vi "Set_Hi-Tec_client.vi"(5 "Row No":i32=1, 6 "Strength (% by volume)":dbl format="%.2f", 7 "Carrier_2 Q (l/min)":dbl=20.0 format="%.2f", 8 "Carrier_1 Q (l/min)":dbl=20.0 format="%.2f", 9 "Mode":enum16{"Control Hi-Tec", "Check Hi-Tec Demands"}(ring)) -> (0 "error out":errorcluster, 1 "Flowrates (kg/min)":dbl[](array[numeric]) format="%.4f")   [LabVIEW 2016]
doc: "This is an example of using features of the VI Server as a client. It shows how you might browse from one or more applications that may be exporting data from one or more data stations. \n\nThe example shows how to query a server for its list of exported VIs, how to get references to the VIs, and how call them with the Call By Reference function."
uses:
  Anemometry/Anemometry Sub Vis/Globals/Preference_global.vi
panel:
  out "Iterations":i32
  in  "Server type":refnum<vi>
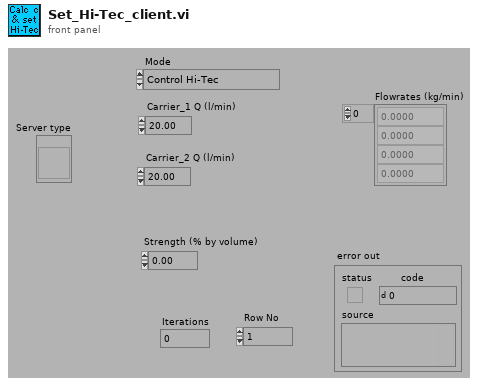
[diagram p1: front panel]
types:
  T1 = typedef "Server_Comms.ctl" = enum16{"Server Link Healthy", "Do Not Link To Server"}
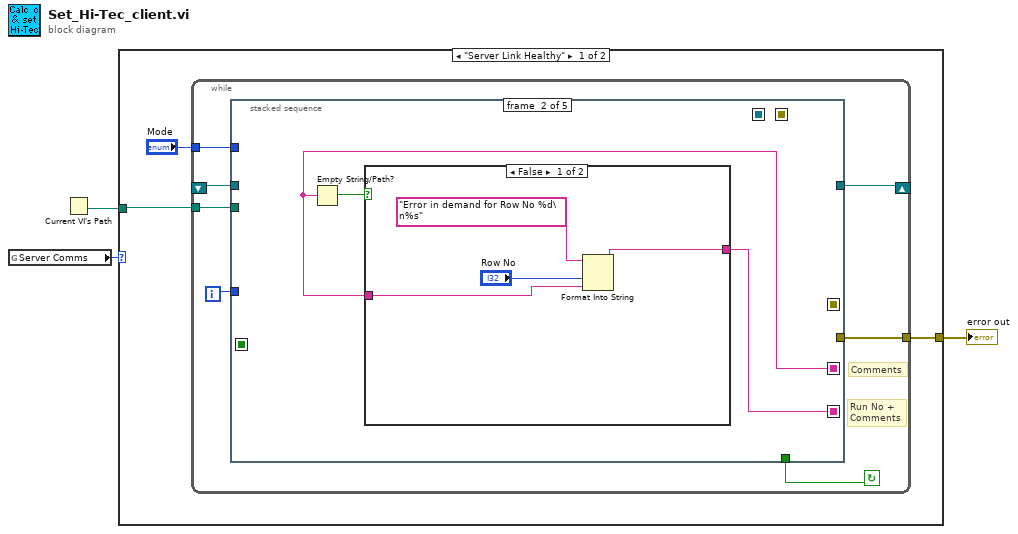
[diagram p0: block diagram]
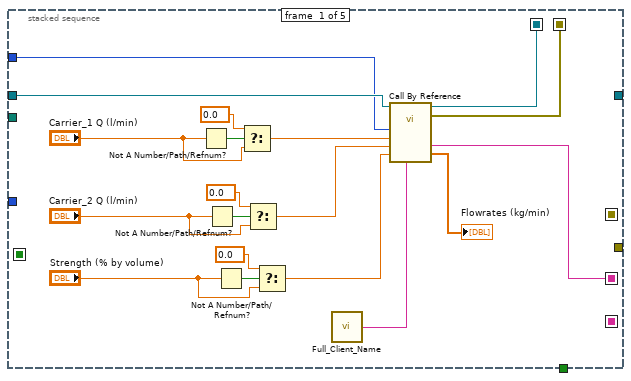
[diagram p2: hidden frame]
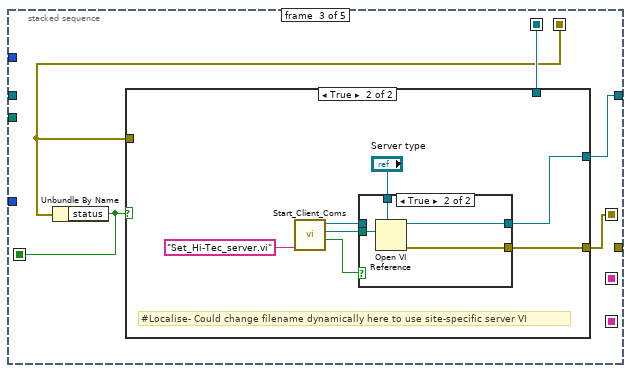
[diagram p4: hidden frame]
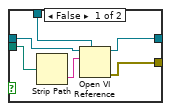
[diagram p6: hidden frame]
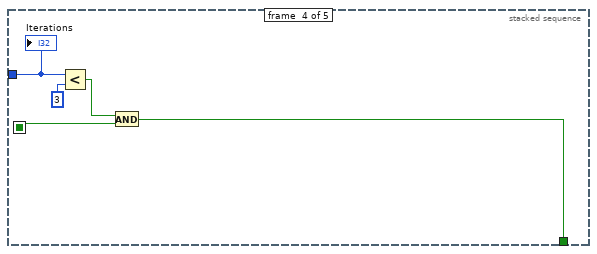
[diagram p7: hidden frame]
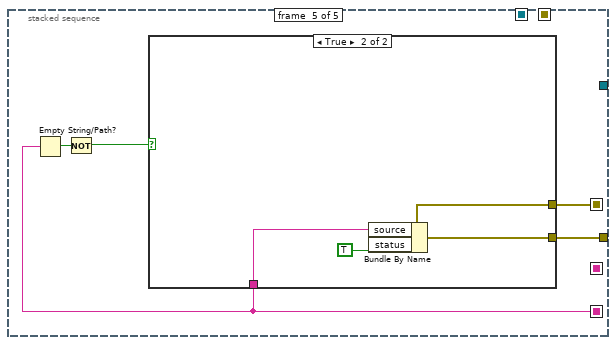
[diagram p8: hidden frame]
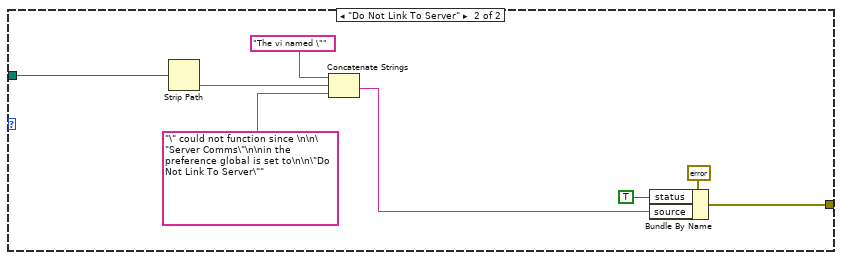
[diagram p10: hidden frame]
diagram:
  n1 = global read "Preference_global.vi" "Server Comms"() -> (w3:T1)
  n2 = Current VI's Path() -> (path=w2:path)
  n3 = case shown="\"Server Link Healthy\"" w3 {
    tunnel: [w6 w81] -> w1
    tunnel: w2 -> [w4 w80]
    frame "Server Link Healthy" {
      n4 = while {
        tunnel: w4 -> [w7]
        tunnel: "Mode" -> [w8]
        tunnel: [w9] -> w6
        shift-left: _ -> [w13]
        shift-right: [w12] -> _
        i -> [w11]
        stop <- w10 continue-if-true
        # "Run No +\nComments"
        # "Comments"
        n5 = stacked-sequence {
          seq-local: [w31 _ _ _ _] -> [_ _ w45 _ _]
          seq-local: [w30 _ _ _ _] -> [_ _ w42 _ _]
          seq-local: [_ _ w43 _ _] -> [_ _ _ w66 _]
          seq-local: [w28 _ _ _ _] -> [_ w34 _ _ _]
          seq-local: [_ w33 _ _ _] -> [_ _ _ _ w72]
          seq-local: [_ _ w41 _ _] -> [_ _ _ _ w74]
          tunnel: w13 -> [w32 _ _ _ _]
          tunnel: [_ _ w44 _ _] -> w12
          tunnel: w11 -> [_ _ _ w69 _]
          tunnel: [_ _ _ w65 _] -> w10
          tunnel: [_ _ _ _ w73] -> w9
          tunnel: w8 -> [w27 _ _ _ _]
          tunnel: w7 -> [_ _ _ _ _]
          frame #0 {
            n6 = Not A Number/Path/Refnum?(number/path/refnum="Carrier_1 Q (l/min)") -> (NaN/Path/Refnum?=w22:bool)
            n7 = Not A Number/Path/Refnum?(number/path/refnum="Carrier_2 Q (l/min)") -> (NaN/Path/Refnum?=w25:bool)
            n8 = Not A Number/Path/Refnum?(number/path/refnum="Strength (% by volume)") -> (NaN/Path/Refnum?=w18:bool)
            n9 = Select(t=0.0, s=w22, f="Carrier_1 Q (l/min)") -> (s? t:f=w16:dbl)
            n10 = Select(t=0.0, s=w25, f="Carrier_2 Q (l/min)") -> (s? t:f=w15:dbl)
            n11 = Select(t=0.0, s=w18, f="Strength (% by volume)") -> (s? t:f=w14:dbl)
            n12 = call "Full_Client_Name.vi"() -> ("Client Name"=w26:string)
            n13 = call-by-ref "?"(reference=w32, "Client Name"=w26, "Strength (% by volume)"=w14, "Carrier_2 Q (l/min)"=w15, "Carrier_1 Q (l/min)"=w16, "Mode"=w27) -> (reference out=w31:refnum<vi>, error out=w30:errorcluster, "Flowrates (kg/min)"=→"Flowrates (kg/min)":dbl[], "Comment"=w28:string)  [unwired: 4 in]
          }
          frame #1 {
            n14 = Empty String/Path?(string/path=w34) -> (empty?=w35:bool)
            n15 = case shown="False" w35 {
              tunnel: w34 -> [w36 w40]
              tunnel: [w38 w40] -> w33
              frame False {
                n16 = Format Into String(format string="Error in demand for Row No %d\n%s" ("Format String"), "Row No", w36) -> (resulting string=w38:string)  [unwired: 2 in, 1 out]
              }
              frame True {
              }
            }
          }
          frame #2 {
            n17 = Unbundle By Name(w42) -> ("status"=w43:bool)
            n18 = case shown="True" w43 {
              tunnel: w45 -> [w47 _]
              tunnel: [w47 w49] -> w44
              tunnel: [w46 w48] -> w41
              tunnel: w42 -> [w46 _]
              frame False {
              }
              frame True {
                # "#Localise- Could change filename dynamically here to use site-specific server VI"
                n19 = call "Start_Client_Coms.vi"("VI name to run on server"="Set_Hi-Tec_server.vi") -> ("LabVIEW application reference"=w53:refnum<vi>, "Checked VI name"=w54:path, "Local Call"=w52:bool)  [unwired: 1 in, 1 out]
                n20 = case shown="True" w52 {
                  tunnel: "Server type" -> [w56 w63]
                  tunnel: w54 -> [w57 w64]
                  tunnel: w53 -> [w55 _]
                  tunnel: [w59 w62] -> w49
                  tunnel: [w58 w61] -> w48
                  frame False {
                    n21 = Strip Path(path=w57) -> (name=w60:string)  [unwired: 1 out]
                    n22 = Open VI Reference(type specifier VI Refnum (for type only)=w56, application reference (local)=w55, vi path=w60) -> (vi reference=w59:refnum<vi>, error out=w58:errorcluster)  [unwired: 1 in, 2 out]
                  }
                  frame True {
                    n23 = Open VI Reference(type specifier VI Refnum (for type only)=w63, vi path=w64) -> (vi reference=w62:refnum<vi>, error out=w61:errorcluster)  [unwired: 1 in, 3 out]
                  }
                }
              }
            }
          }
          frame #3 {
            n24 = Less?(x=w69, y=3) -> (x < y?=w67:bool)
            n25 = And(x=w67, y=w66) -> (x .and. y?=w65:bool)
            "Iterations" <- w69
          }
          frame #4 {
            n26 = Empty String/Path?(string/path=w72) -> (empty?=w71:bool)
            n27 = Not(x=w71) -> (.not. x?=w70:bool)
            n28 = case shown="True" w70 {
              tunnel: w74 -> [w75 w79]
              tunnel: w72 -> [_ w76]
              tunnel: [w75 w78] -> w73
              frame False {
              }
              frame True {
                n29 = Bundle By Name(cluster=w79, "source"=w76, "status"=TRUE ("Bundle Element")) -> (w78:errorcluster)
              }
            }
          }
        }
      }
    }
    frame "Do Not Link To Server" {
      n30 = Strip Path(path=w80) -> (name=w86:string)  [unwired: 1 out]
      n31 = Concatenate Strings("The vi named \"", w86, "\" could not function since \n\n\"Server Comms\"\n\nin the preference global is set to\n\n\"Do Not Link To Server\"") -> (w83:string)
      n32 = Bundle By Name(cluster=errorcluster {"status"=FALSE, "code"=0, "source"=""}, "status"=TRUE ("Bundle Element"), "source"=w83) -> (w81:errorcluster)
    }
  }
  "error out" <- w1
